vi "Class Loading Result.vi"(0 "Test Caller Actor in":refnum<class "Test Caller Actor.lvclass">, 5 "Classes Map":T1, 7 "Class Array":refnum<class>[](array[class]), 9 "Class Names":string[](array[string]), 11 "error in (no error)":errorcluster) -> (4 "Test Caller Actor out":refnum<class "Test Caller Actor.lvclass">, 15 "error out":errorcluster)   [LabVIEW 2023, in "Test Caller Actor.lvlib" / "Test Caller Actor.lvclass"]
uses:
  Test Caller Actor.lvclass
  Class Loader/Class Loader/Classes Map.ctl
  Load Complete Data.ctl
  Test Caller Actor.lvclass/Test Caller Actor.ctl
  Class Loader/Class Loader/Class Loader.lvclass
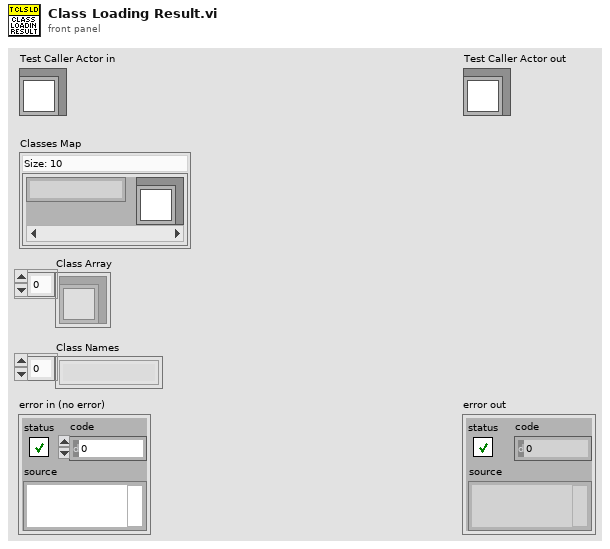
[diagram p1: front panel]
types:
  T1 = typedef "Class Loader.lvlib/Class Loader.lvclass/Classes Map.ctl" = map{string, refnum<class>}
  T2 = typedef "Test Caller Actor.lvlib/Test Caller Actor.lvclass/Load Complete Data.ctl" = cluster{"Load Complete":bool, "Class Names":string[]}
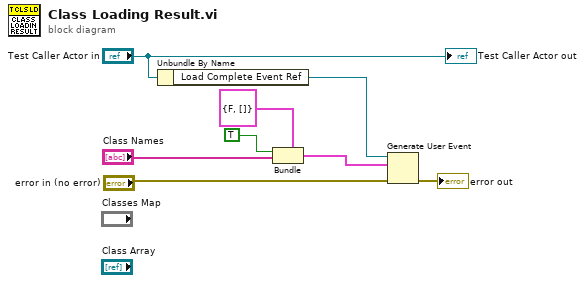
[diagram p0: block diagram]
diagram:
  n1 = Unbundle By Name("Test Caller Actor in") -> ("Load Complete Event Ref"=w6:refnum<user-event>)
  n2 = Bundle(cluster=T2 {"Load Complete"=FALSE, "Class Names"=[]} ("event data"), "Load Complete"=TRUE, "Class Names"="Class Names") -> (w1:T2)
  n3 = Generate User Event(user event=w6, event data cluster=w1, error in="error in (no error)") -> (error out=→"error out":errorcluster)  [unwired: 1 in, 1 out]
  "Test Caller Actor out" <- "Test Caller Actor in"
